vi "Set Level.vi"(6 "Output Channel":T1, 8 "error in (no error)":errorcluster, 9 "Slew (V/s)":dbl, 10 "Level (V)":dbl, 11 "Inst.RP100 in":refnum<class "Inst.RP100.lvclass">) -> (0 "error out":errorcluster, 3 "Inst.RP100 out":refnum<class "Inst.RP100.lvclass">)   [LabVIEW 2019, in "Inst.RP100.lvlib" / "Inst.RP100.lvclass"]
doc: "Set the output <b>Level</b> with <b>Slew</b> rate on the selected <b>Output Channel</b>"
uses:
  Inst.RP100.lvclass
  Typedefs/Channel--Num.ctl
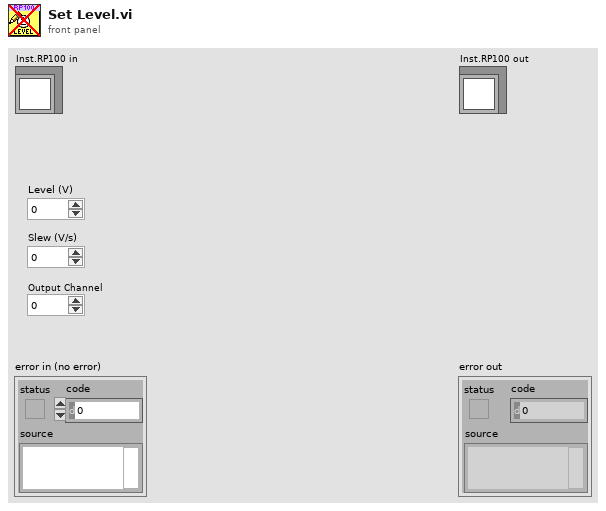
[diagram p1: front panel]
types:
  T1 = typedef "Inst.RP100.lvlib/Inst.RP100.lvclass/Channel--Num.ctl" = i32
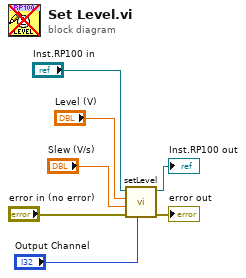
[diagram p0: block diagram]
diagram:
  n1 = call-dynamic "setLevel.vi"("Output Channel"="Output Channel", "error in (no error)"="error in (no error)", "Slew (V/s)"="Slew (V/s)", "Level (V)"="Level (V)", "Inst.RP100 in"="Inst.RP100 in") -> ("error out"=→"error out":errorcluster, "Inst.RP100 out"=→"Inst.RP100 out":refnum<class "Inst.RP100.lvclass">)  [unwired: 5 in]
